vi "set_subjectID.vi"() -> (2 "subject_id":string)   [LabVIEW 2020]
uses:
  <vilib>/Utility/error.llb/Trim Whitespace One-Sided.vi
panel:
  in  "save_return":bool
  in  "subject_id_in":string
  # "Enter Patient ID(can not be empty)"
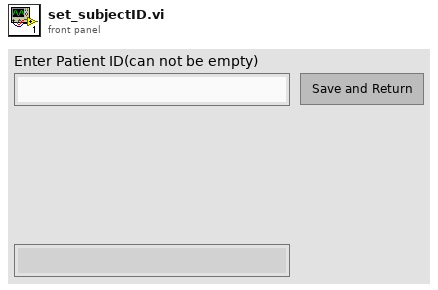
[diagram p1: front panel]
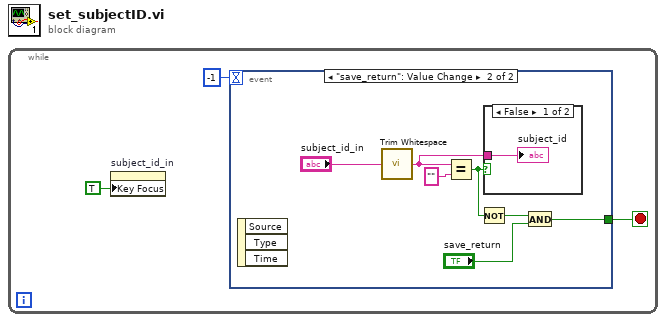
[diagram p0: block diagram]
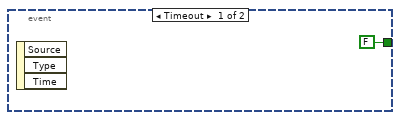
[diagram p2: hidden frame]
diagram:
  n1 = while {
    stop <- w3 stop-if-true
    n2 = property on="subject_id_in" class="Str"("Key Focus"=TRUE) -> ()  [unwired: 2 in, 2 out]
    n3 = event shown="[1] \"save_return\": Value Change" {
      selector: _ -> [_ _]
      dyn-events: _ -> [_ _]
      timeout: -1 -> [_ _]
      tunnel: [FALSE w5] -> w3
      event Timeout {
        n4 = event-data() -> ()  [unwired: 1 in, 3 out]
      }
      event "save_return": Value Change {
        n5 = event-data() -> ()  [unwired: 1 in, 3 out]
        n6 = call <vilib>:"Trim Whitespace.vi"("string"="subject_id_in") -> ("trimmed string"=w8:string)  [unwired: 1 in]
        n7 = Equal?(x=w8, y="") -> (x = y?=w11:bool)
        n8 = Not(x=w11) -> (.not. x?=w10:bool)
        n9 = case shown="False" w11 {
          tunnel: w8 -> [w12 _]
          frame False {
            "subject_id" <- w12
          }
          frame True {
          }
        }
        n10 = And(x=w10, y="save_return") -> (x .and. y?=w5:bool)
      }
    }
  }
